vi "求角度.vi"(7 "Line form":enum16{"Line", "Two Point"}(ring)=enum."Two Point", 9 "Point 2":cluster{"X":sgl, "Y":sgl}, 10 "Point 1":cluster{"X":sgl, "Y":sgl}, 11 "Line":T1) -> (2 "rotate radius":sgl, 3 "rotate":sgl)   [LabVIEW 2015]
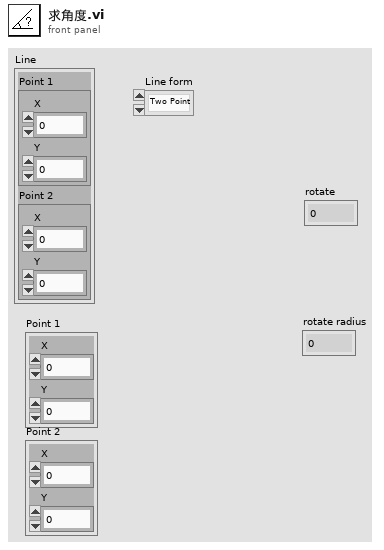
[diagram p1: front panel]
types:
  T1 = cluster{"Point 1":cluster{"X":sgl, "Y":sgl}, "Point 2":cluster{"X":sgl, "Y":sgl}}
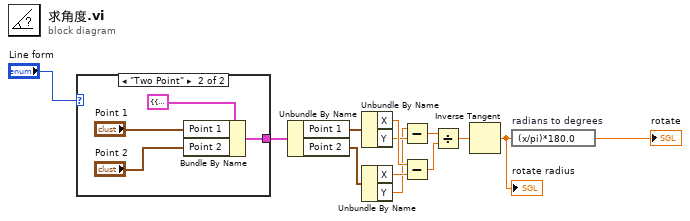
[diagram p0: block diagram]
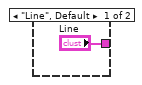
[diagram p2: hidden frame]
diagram:
  n1 = case shown="\"Two Point\"" "Line form" {
    tunnel: ["Line" w15] -> w1
    frame "Line", Default {
    }
    frame "Two Point" {
      n2 = Bundle By Name(cluster=T1 {"Point 1"={"X"=0.0, "Y"=0.0}, "Point 2"={"X"=0.0, "Y"=0.0}} ("Line"), "Point 1"="Point 1", "Point 2"="Point 2") -> (w15:T1)
    }
  }
  n3 = Unbundle By Name(w1) -> ("Point 1"=w5:cluster{"X":sgl, "Y":sgl}, "Point 2"=w6:cluster{"X":sgl, "Y":sgl})
  n4 = Unbundle By Name(w5) -> ("X"=w13:sgl, "Y"=w11:sgl)
  n5 = Unbundle By Name(w6) -> ("X"=w12:sgl, "Y"=w10:sgl)
  n6 = Subtract(x=w10, y=w11) -> (x-y=w8:sgl)
  n7 = Subtract(x=w13, y=w12) -> (x-y=w9:sgl)
  n8 = Divide(x=w8, y=w9) -> (x/y=w7:sgl)
  n9 = Inverse Tangent(1:w7) -> (0:w3:sgl)
  "rotate radius" <- w3
  n10 = expression code="(x/pi)*180.0" "radians to degrees"(w3) -> (→"rotate":sgl)
